vi "VersionConversionData.vi"(8 "Error In":errorcluster, 10 "Version In":string) -> (0 "Error Out":errorcluster, 2 "Version Out":string)   [LabVIEW 2023]
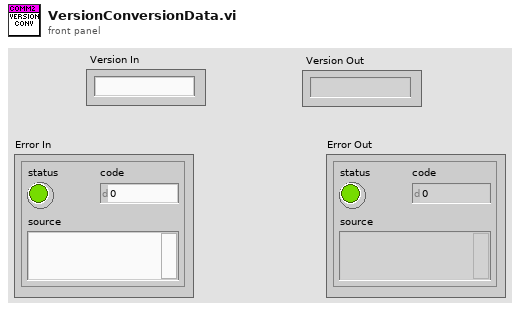
[diagram p1: front panel]
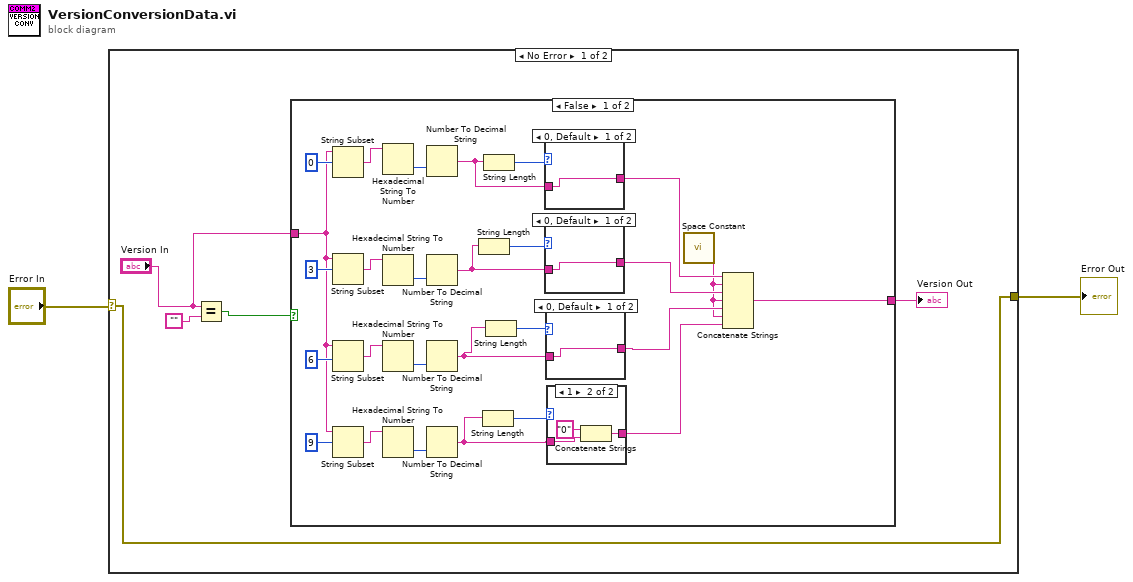
[diagram p0: block diagram]
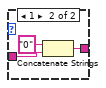
[diagram p3: hidden frame]
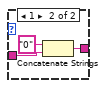
[diagram p4: hidden frame]
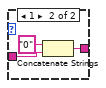
[diagram p5: hidden frame]
diagram:
  n1 = case shown="No Error" "Error In" {
    selector: "Error In" -> [w3 w52]
    tunnel: [w3 w52] -> w1
    frame No Error {
      n2 = Equal?(x="Version In", y="") -> (x = y?=w6:bool)
      n3 = case shown="False" w6 {
        tunnel: "Version In" -> [w9 w51]
        tunnel: [w8 w51] -> w4
        frame False {
          n4 = String Subset(string=w9, offset (0)=0 ("length (rest)")) -> (substring=w32:string)  [unwired: 1 in]
          n5 = String Subset(string=w9, offset (0)=3 ("length (rest)")) -> (substring=w31:string)  [unwired: 1 in]
          n6 = String Subset(string=w9, offset (0)=6) -> (substring=w28:string)  [unwired: 1 in]
          n7 = String Subset(string=w9, offset (0)=9) -> (substring=w27:string)  [unwired: 1 in]
          n8 = Hexadecimal String To Number(string=w32) -> (number=w30:u32)  [unwired: 2 in, 1 out]
          n9 = Hexadecimal String To Number(string=w31) -> (number=w29:u32)  [unwired: 2 in, 1 out]
          n10 = Hexadecimal String To Number(string=w28) -> (number=w26:u32)  [unwired: 2 in, 1 out]
          n11 = Hexadecimal String To Number(string=w27) -> (number=w23:u32)  [unwired: 2 in, 1 out]
          n12 = Number To Decimal String(number=w30) -> (decimal integer string=w21:string)  [unwired: 1 in]
          n13 = Number To Decimal String(number=w29) -> (decimal integer string=w15:string)  [unwired: 1 in]
          n14 = Number To Decimal String(number=w26) -> (decimal integer string=w17:string)  [unwired: 1 in]
          n15 = Number To Decimal String(number=w23) -> (decimal integer string=w18:string)  [unwired: 1 in]
          n16 = String Length(string=w15) -> (length=w16:i32)
          n17 = String Length(string=w18) -> (length=w19:i32)
          n18 = String Length(string=w21) -> (length=w22:i32)
          n19 = String Length(string=w17) -> (length=w20:i32)
          n20 = case shown="0, Default" w22 {
            tunnel: w21 -> [w47 w49]
            tunnel: [w47 w48] -> w14
            frame 0, Default {
            }
            frame 1 {
              n21 = Concatenate Strings("0" ("string"), w49) -> (w48:string)
            }
          }
          n22 = case shown="0, Default" w16 {
            tunnel: [w43 w45] -> w13
            tunnel: w15 -> [w43 w44]
            frame 0, Default {
            }
            frame 1 {
              n23 = Concatenate Strings("0" ("string"), w44) -> (w45:string)
            }
          }
          n24 = case shown="0, Default" w20 {
            tunnel: w17 -> [w39 w41]
            tunnel: [w39 w40] -> w12
            frame 0, Default {
            }
            frame 1 {
              n25 = Concatenate Strings("0" ("string"), w41) -> (w40:string)
            }
          }
          n26 = case shown="1" w19 {
            tunnel: w18 -> [w35 w37]
            tunnel: [w35 w36] -> w11
            frame 0, Default {
            }
            frame 1 {
              n27 = Concatenate Strings("0" ("string"), w37) -> (w36:string)
            }
          }
          n28 = call <vilib>:"Space Constant.vi"() -> ("String"=w10:string)
          n29 = Concatenate Strings(w14, w10, w13, w10, w12, w10, w11) -> (w8:string)
        }
        frame True {
        }
      }
      "Version Out" <- w4
    }
    frame Error {
    }
  }
  "Error Out" <- w1
